vi "Wait Notification.vi"(8 "error in (no error)":errorcluster, 9 "Timeout":i32, 11 "SEQ I64 in":refnum<class "SEQ I64.lvclass">) -> (0 "error out":errorcluster, 1 "Timeout?":bool, 2 "Notification":variant, 3 "SEQ I64 out":refnum<class "SEQ I64.lvclass">)   [LabVIEW 2024, in "SEQ I64.lvclass"]
uses:
  SEQ I64.lvclass
  SEQ I64.lvclass/SEQ I64.ctl
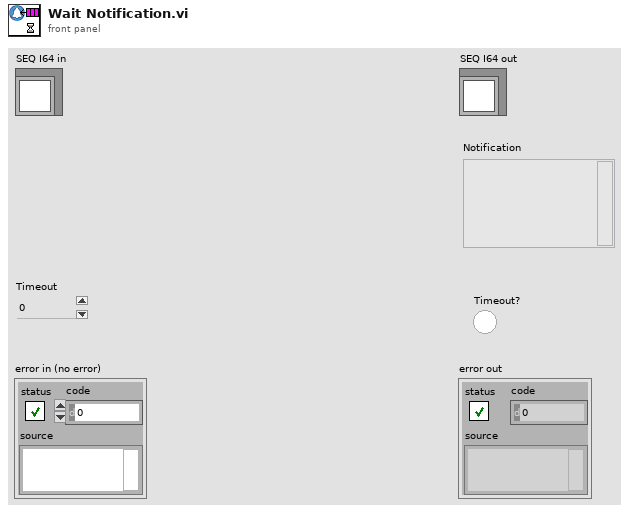
[diagram p1: front panel]
types:
  T1 = typedef "Control 2.ctl" = refnum<queue>
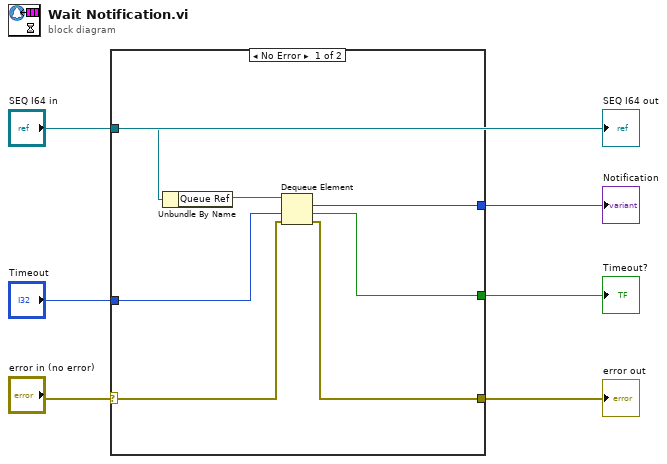
[diagram p0: block diagram]
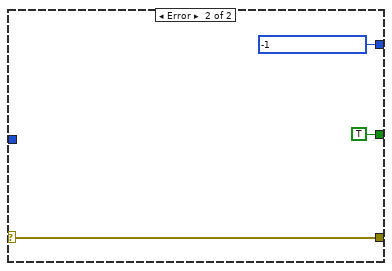
[diagram p2: hidden frame]
diagram:
  n1 = case shown="No Error" "error in (no error)" {
    selector: "error in (no error)" -> [w8 w15]
    tunnel: "SEQ I64 in" -> [w13 _]
    tunnel: "Timeout" -> [w11 _]
    tunnel: [w10 i64 -1] -> w4
    tunnel: [w9 TRUE ("timed out?")] -> w3
    tunnel: [w7 w15] -> w1
    frame No Error {
      n2 = Unbundle By Name(w13) -> ("Queue Ref"=w12:T1)
      n3 = Dequeue Element(queue=w12, timeout in ms (-1)=w11, error in (no error)=w8) -> (element=w10:i64, timed out?=w9:bool, error out=w7:errorcluster)  [unwired: 1 out]
    }
    frame Error {
    }
  }
  "error out" <- w1
  "Notification" <- w4
  "Timeout?" <- w3
  "SEQ I64 out" <- "SEQ I64 in"
